vi "Send-status.vi"(8 "error in (no error)":errorcluster, 10 "Status":T1, 11 "Client in":T2) -> (0 "error out":errorcluster, 3 "Client out":T2)   [LabVIEW 2013, in "CameraVision.lvlib" / "CV-Client.lvclass"]
doc: "Send a message to the specified list of receivers.\nThe message is added to the back of the server message queue for processing.\nThe message needs to be created beforehand, either manually or through the 'Create-message' function and any specific contents need to be pre-configured. This function takes care of the sender and time information.\nThe receivers must be provided as an array. Each receiver entry can be composed in two ways: either '<module type>' to send to all active clients of the specified type, or '<module type><module ID>' to send to a specific client. Optionally the special client types 'All' or 'Server' can be used to send the message to all active clients (server excluded) or to the server, respectively."
uses:
  CV-Client.lvclass
  Object-reference.ctl
  Application-states.ctl
  Supported-modules.ctl
  SA-SLMAPI/Sources/Send-status/Send-status.lvclass
  CV-Main.lvclass
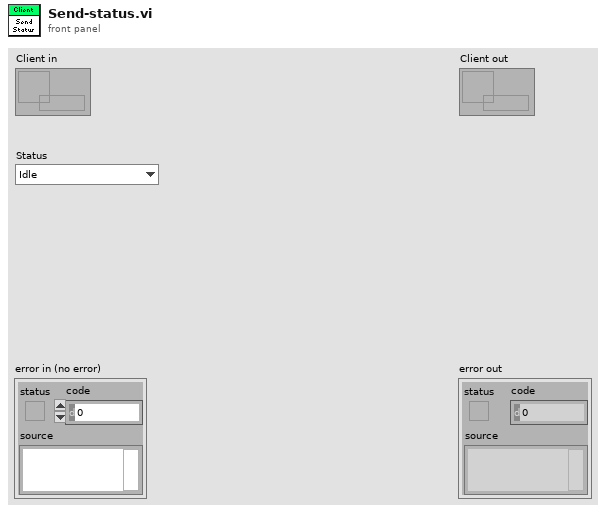
[diagram p1: front panel]
types:
  T1 = typedef "CameraVision.lvlib/CV-Main.lvclass/Application-states.ctl" = enum16{"Idle", "Initialized", "Configured", "Activated", "Started", "Stopped", "Reset", "Error", "Exited"}
  T2 = typedef "CameraVision.lvlib/CV-Client.lvclass/Object-reference.ctl" = refnum<data-value>
  T3 = typedef "CameraVision.lvlib/CV-Client.lvclass/Supported-modules.ctl" = enum16{"Server", "All", "SLMControl", "PowderDeposition", "StrategyParser", "CameraVision", "MaterialCharacterization", "StatusMonitor", "SLMSimulation", "LaserCharacterization"}
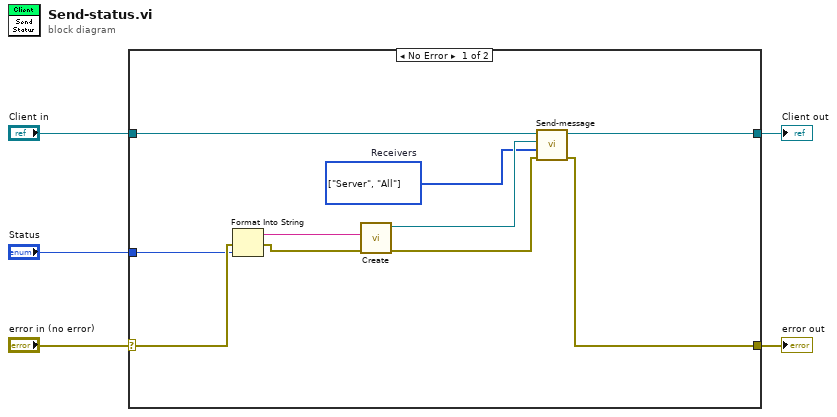
[diagram p0: block diagram]
diagram:
  n1 = case shown="No Error" "error in (no error)" {
    selector: "error in (no error)" -> [w7 w17]
    tunnel: [w8 w17] -> w4
    tunnel: [w9 w16] -> w2
    tunnel: "Client in" -> [w10 w16]
    tunnel: "Status" -> [w6 _]
    frame No Error {
      w11 = T3[] [enum."Server", enum."All"] items=["Server", "All", "SLMControl", "PowderDeposition", "StrategyParser", "CameraVision", "MaterialCharacterization", "StatusMonitor", "SLMSimulation", "LaserCharacterization"]  # Receivers
      n2 = Format Into String(error in=w7, w6) -> (resulting string=w15:string, error out=w12:errorcluster)  [unwired: 2 in]
      n3 = call "Create.vi"("error in (no error)"=w12, "Status"=w15) -> ("error out"=w13:errorcluster, "Send-status out"=w14:refnum<class "Send-status.lvclass">)  [unwired: 8 in]
      n4 = call "Send-message.vi"("error in (no error)"=w13, "Receivers"=w11, "Message"=w14, "Client in"=w10) -> ("error out"=w8:errorcluster, "Client out"=w9:T2)  [unwired: 6 in]
    }
    frame Error {
    }
  }
  "error out" <- w4
  "Client out" <- w2
